vi "ProjectVI.vi"() -> ()   [LabVIEW 2024]
panel:
  out "Waveform Chart":dynamicdata(graph)
  in  "stop (F)":bool
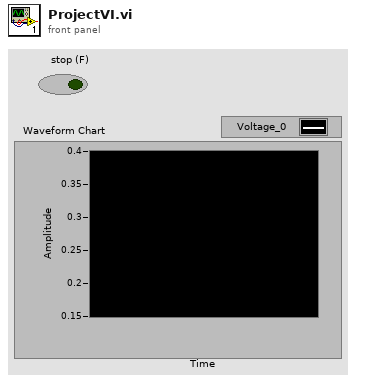
[diagram p1: front panel]
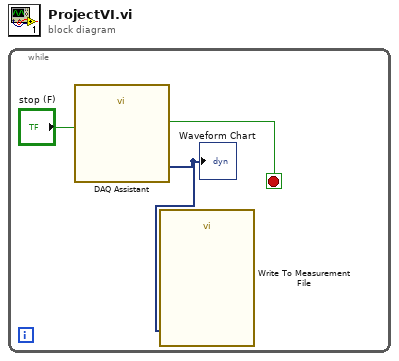
[diagram p0: block diagram]
diagram:
  n1 = while {
    stop <- w2 stop-if-true
    n2 = call "DAQ Assistant"("stop (F)"="stop (F)") -> ("data"=w1:dynamicdata, "stopped"=w2:bool)  [unwired: 15 in, 2 out]
    "Waveform Chart" <- w1
    n3 = call "Write To Measurement File"("Signals"=w1) -> ()  [unwired: 16 in, 3 out]
  }
